vi "APS get task msg.vi"(7 "CharArr":string, 8 "error in (no error)":errorcluster caption="错误输入（无错误）", 9 "ActualSize":u16, 10 "QueueSts":u16, 11 "Board_ID":i32) -> (0 "error out":errorcluster caption="错误输出", 1 "ActualSize out":u16, 2 "QueueSts out":u16, 3 "function return":i32, 5 "CharArr out":string)   [LabVIEW 2011, in "APS168.lvlib"]
doc: "I32 FNTYPE APS_get_task_msg( I32 Board_ID, U16 *QueueSts, U16 *ActualSize, U8 *CharArr );"
uses:
  APS168.lvlib
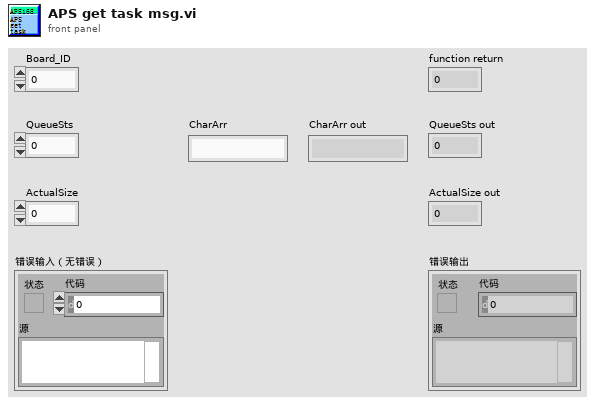
[diagram p1: front panel]
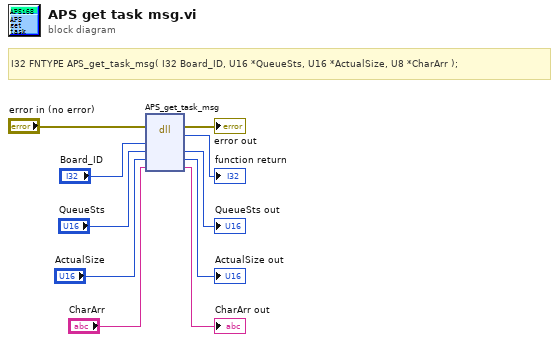
[diagram p0: block diagram]
diagram:
  # "I32 FNTYPE APS_get_task_msg( I32 Board_ID, U16 *QueueSts, U16 *ActualSize, U8 *CharArr );"
  n1 = dll-call lib="PTH1Labs E软件ADLINK 204CAPS_1_7_1_LIB line 连续运动204APS168.*" fn="APS_get_task_msg"(error in="error in (no error)", "Board_ID"="Board_ID", "QueueSts"="QueueSts", "ActualSize"="ActualSize", "CharArr"="CharArr") -> (error out=→"error out":errorcluster, →"function return":i32, "QueueSts"=→"QueueSts out":u16, "ActualSize"=→"ActualSize out":u16, "CharArr"=→"CharArr out":string)  [unwired: 3 in, 1 out]
